vi "Rohde & Schwarz VNA Set Cal Off.vi"(7 "Rohde & Schwarz VNA":T1, 8 "error in (no error)":errorcluster, 11 "VISA Resource Name":refnum<visa-resource-name>) -> (0 "error out":errorcluster {"code" format="%.0x"}, 3 "dup VISA Resource Name":refnum<visa-resource-name>)   [LabVIEW 2011]
doc: "This Vi for the HP8753B Network Analyzer is used to set averaging, smoothing, and the IF bandwidth."
uses:
  TypeDefs/Rohde & Schwarz VNA Instrument Info.ctl
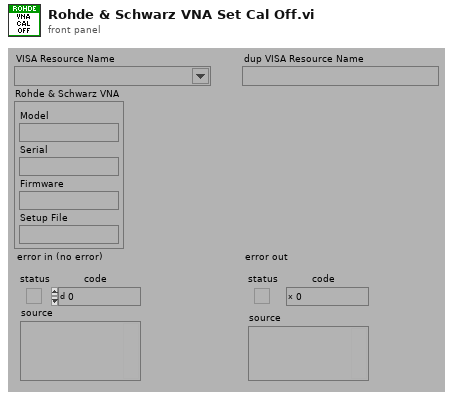
[diagram p1: front panel]
types:
  T1 = typedef "Rohde & Schwarz VNA Instrument Info.ctl" = cluster{"Model":string, "Serial":string, "Firmware":string, "Setup File":string}
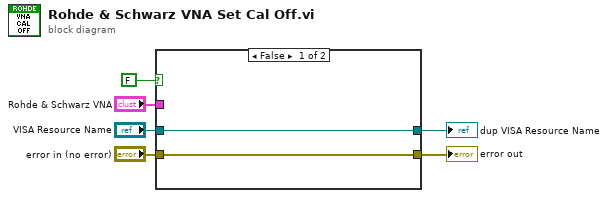
[diagram p0: block diagram]
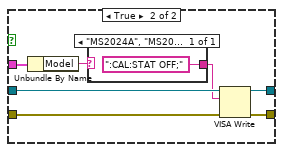
[diagram p2: hidden frame]
diagram:
  n1 = case shown="False" FALSE {
    tunnel: "VISA Resource Name" -> [w8 w15]
    tunnel: "error in (no error)" -> [w7 w14]
    tunnel: [w7 w13] -> w4
    tunnel: [w8 w12] -> w3
    tunnel: "Rohde & Schwarz VNA" -> [_ w10]
    frame False {
    }
    frame True {
      n2 = Unbundle By Name(w10) -> ("Model"=w9:string)
      n3 = case shown="\"MS2024A\", \"MS2026A\", Default" w9 {
        tunnel: [":CAL:STAT OFF;"] -> w11
        frame "MS2024A", "MS2026A", Default {
        }
      }
      n4 = VISA Write(VISA resource name=w15, write buffer=w11, error in (no error)=w14) -> (VISA resource name out=w12:refnum<visa-resource-name>, error out=w13:errorcluster)  [unwired: 1 out]
    }
  }
  "error out" <- w4
  "dup VISA Resource Name" <- w3
